vi "q2w4.vi"() -> ()   [LabVIEW 2021]
panel:
  out "Waveform Graph":dynamicdata(graph)
  out "THD":dbl
  out "PEAK TO PEAK":dbl
  out "RMS":dbl
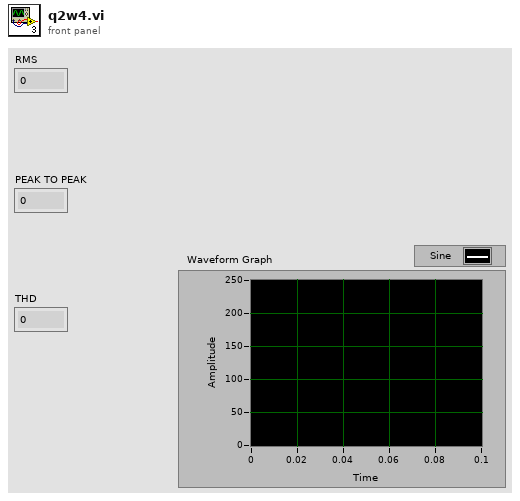
[diagram p1: front panel]
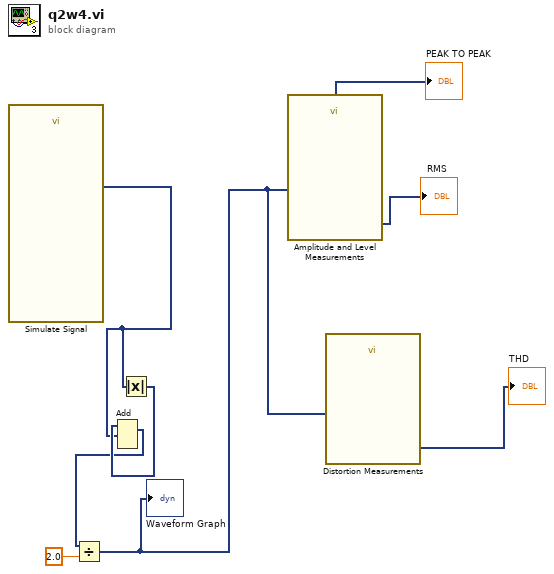
[diagram p0: block diagram]
diagram:
  n1 = call "Simulate Signal"() -> ("Sine"=w5:dynamicdata)  [unwired: 14 in, 1 out]
  n2 = Absolute Value(x=w5) -> (abs(x)=w6:dynamicdata)
  n3 = Add(1:w5, 2:w6) -> (0:w3:dynamicdata)  [unwired: 1 in, 1 out]
  n4 = Divide(x=w3, y=2.0) -> (x/y=w1:dynamicdata)
  "Waveform Graph" <- w1
  n5 = call "Amplitude and Level Measurements"("Signals"=w1) -> ("RMS"=→"RMS":dynamicdata, "Peak to Peak"=→"PEAK TO PEAK":dynamicdata)  [unwired: 12 in, 1 out]
  n6 = call "Distortion Measurements"("Signals"=w1) -> ("THD"=→"THD":dynamicdata)  [unwired: 8 in, 2 out]
